vi "SetWavelength.vi"(8 "error in (no error)":errorcluster, 10 "Wavelength, nm":dbl=620.0, 11 "MC":refnum<class "MC.lvclass">) -> (0 "error out":errorcluster, 3 "MC out":refnum<class "MC.lvclass">)   [LabVIEW 2017, in "MC.lvclass"]
doc: "---------------------------------------------------------------\nJKI State Machine Objects™\nhttp://jki.net/state-machine-objects/\nCopyright (C) 2005-2015, JKI <info@jki.net>\nALL RIGHTS RESERVEDJKI State Machine Objects (SMO) 1.0.0.5\nJKI - JKI\nCopyright (c) 2016, JKI"
uses:
  MC.lvclass
  Typedefs/PrivateEvents--MC.SetWavelength.ctl
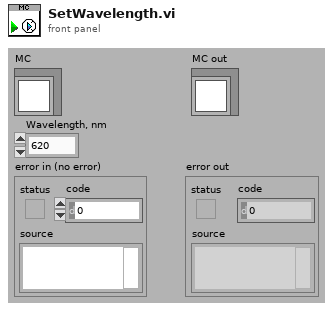
[diagram p1: front panel]
types:
  T1 = typedef "MC.lvclass/PrivateEvents--MC.SetWavelength.ctl" = cluster{"Wavelength, nm":dbl}
  T2 = typedef "MC.lvclass/PrivateEvents--Cluster.ctl" = cluster{"New Value":refnum<user-event>, "SetWavelength":refnum<user-event>}
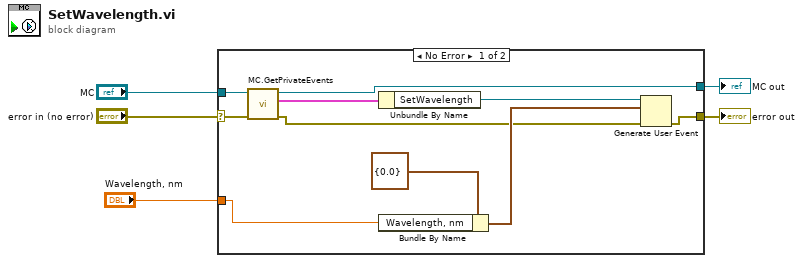
[diagram p0: block diagram]
diagram:
  n1 = case shown="No Error" "error in (no error)" {
    selector: "error in (no error)" -> [w14 w17]
    tunnel: [w7 w17] -> w5
    tunnel: "MC" -> [w15 w16]
    tunnel: "Wavelength, nm" -> [w11 _]
    tunnel: [w6 w16] -> w1
    frame No Error {
      n2 = call "MC.GetPrivateEvents.vi"("error in (no error)"=w14, "MC"=w15) -> ("error out"=w8:errorcluster, "Private Events"=w13:T2, "MC out"=w6:refnum<class "MC.lvclass">)  [unwired: 7 in]
      n3 = Unbundle By Name(w13) -> ("SetWavelength"=w10:refnum<user-event>)
      n4 = Bundle By Name(cluster=T1 {"Wavelength, nm"=0.0} ("SetWavelength"), "Wavelength, nm"=w11) -> (w9:T1)
      n5 = Generate User Event(user event=w10, event data cluster=w9, error in=w8) -> (error out=w7:errorcluster)  [unwired: 1 in, 1 out]
    }
    frame Error {
    }
  }
  "error out" <- w5
  "MC out" <- w1
